vi "Log to Host.vi"(8 "error in":errorcluster, 10 "Detail":string, 11 "MSS Target Actor in":refnum<class "MSS Target Actor.lvclass">) -> (0 "error out":errorcluster, 3 "MSS Target Actor out":refnum<class "MSS Target Actor.lvclass">)   [LabVIEW 2023, in "MSS Target Actor.lvlib" / "MSS Target Actor.lvclass"]
uses:
  MSS Target Actor.lvclass
  MAL/Study/Study Actor/IStudy Actor Messages/Log Target Msg/Log Target Msg.lvclass
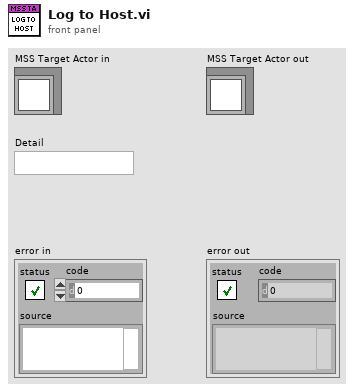
[diagram p1: front panel]
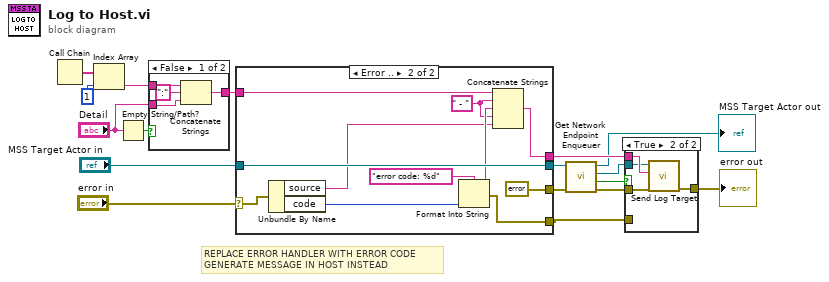
[diagram p0: block diagram]
diagram:
  # "REPLACE ERROR HANDLER WITH ERROR CODE\nGENERATE MESSAGE IN HOST INSTEAD"
  n1 = Call Chain() -> (call chain=w6:string[])
  n2 = Index Array(array=w6, index=1) -> (element=w4:string)
  n3 = Empty String/Path?(string/path="Detail") -> (empty?=w3:bool)
  n4 = case shown="False" w3 {
    tunnel: w4 -> [w21 w22]
    tunnel: "Detail" -> [w19 _]
    tunnel: [w18 w22] -> w1
    frame False {
      n5 = Concatenate Strings(w21, ":" ("string"), w19) -> (w18:string)
    }
    frame True {
    }
  }
  n6 = case shown="Error .." "error in" {
    selector: "error in" -> [w25 w31]
    tunnel: "MSS Target Actor in" -> [w24 w36]
    tunnel: [w24 w36] -> w12
    tunnel: [w23 w35] -> w11
    tunnel: [w25 errorcluster {"status"=FALSE, "code"=0, "source"=""} ("error in (no error)")] -> w9
    tunnel: [_ w28] -> w8
    tunnel: w1 -> [w23 w33]
    frame No Error {
    }
    frame Error {
      w27 = " - " ("string")
      n7 = Unbundle By Name(w31) -> ("source"=w26:string, "code"=w32:i32)
      n8 = Format Into String(format string="error code: %d", w32) -> (resulting string=w29:string, error out=w28:errorcluster)  [unwired: 2 in]
      n9 = Concatenate Strings(w33, w27, w29, w27, w26) -> (w35:string)
    }
  }
  n10 = call "Get Network Endpoint Enqueuer.vi"("error in"=w9, "MSS Target Actor in"=w12) -> ("error out"=w16:errorcluster, "Connected?"=w15:bool, "Enqueuer"=w10:refnum<class "Message Enqueuer.lvclass">, "MSS Target Actor out"=→"MSS Target Actor out":refnum<class "MSS Target Actor.lvclass">)  [unwired: 6 in]
  n11 = case shown="True" w15 {
    tunnel: w16 -> [_ w38]
    tunnel: w11 -> [_ w41]
    tunnel: [w37 w40] -> w17
    tunnel: w10 -> [_ w39]
    tunnel: w8 -> [w37 _]
    frame False {
    }
    frame True {
      n12 = call "Send Log Target.vi"("error in (no error)"=w38, "Entry"=w41, "Message Enqueuer"=w39) -> ("error out"=w40:errorcluster)  [unwired: 7 in, 1 out]
    }
  }
  "error out" <- w17
